vi "Read TC_PID.vi"(0 "read buffer":string, 11 "Error In":errorcluster) -> (4 "Temp (C)":dbl, 6 "On/Off Actual":bool, 8 "On/Off Set":bool, 10 "Temp Set Point (C)":i32, 13 "PID values":dbl[](array[numeric]), 14 "PWM":i32, 15 "Error Out":errorcluster)   [LabVIEW 2015]
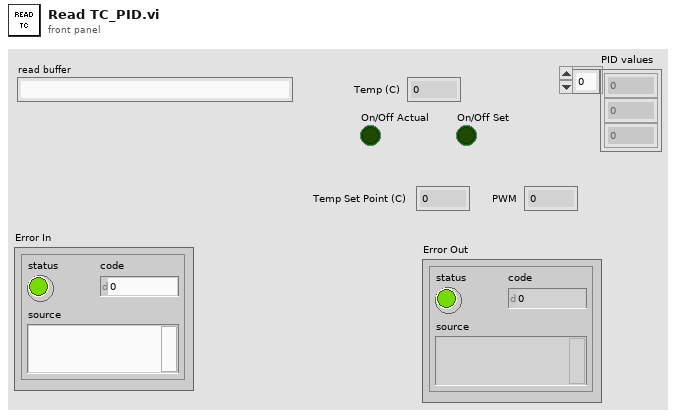
[diagram p1: front panel]
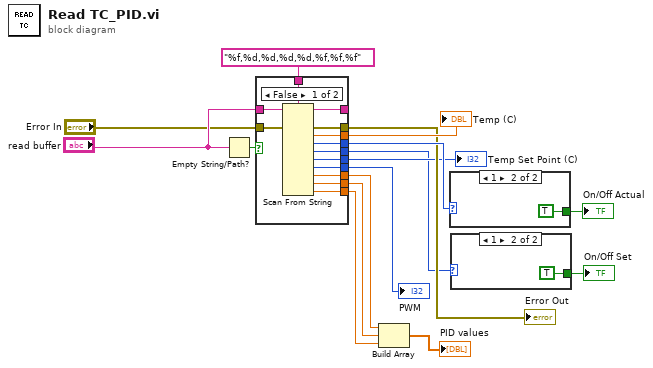
[diagram p0: block diagram]
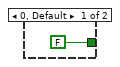
[diagram p2: hidden frame]
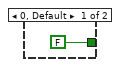
[diagram p3: hidden frame]
diagram:
  n1 = Empty String/Path?(string/path="read buffer") -> (empty?=w15:bool)
  n2 = case shown="False" w15 {
    tunnel: "read buffer" -> [w29 w31]
    tunnel: "%f,%d,%d,%d,%d,%f,%f,%f" ("format string") -> [w28 _]
    tunnel: [w27 w31] -> _
    tunnel: [w26 _] -> w13
    tunnel: [w25 _] -> w6
    tunnel: [w24 _] -> w12
    tunnel: [w23 w30] -> w10
    tunnel: "Error In" -> [w22 w30]
    tunnel: [w21 _] -> w7
    tunnel: [w20 _] -> w5
    tunnel: [w19 _] -> w4
    tunnel: [w18 _] -> w3
    tunnel: [w17 _] -> w2
    frame False {
      n3 = Scan From String(format string=w28, input string=w29, error in=w22) -> (remaining string=w27:string, error out=w23:errorcluster, output 1=w26:dbl, output 2=w24:i32, output 3=w25:i32, output 4=w21:i32, output 5=w20:i32, output 6=w19:dbl, output 7=w18:dbl, output 8=w17:dbl)  [unwired: 9 in, 1 out]
    }
    frame True {
    }
  }
  "Temp (C)" <- w13
  "Temp Set Point (C)" <- w7
  "Error Out" <- w10
  "PWM" <- w5
  n4 = Build Array(w4, w3, w2) -> (→"PID values":dbl[])
  n5 = case shown="1" w12 {
    tunnel: [FALSE TRUE] -> w11
    frame 0, Default {
    }
    frame 1 {
    }
  }
  "On/Off Actual" <- w11
  n6 = case shown="1" w6 {
    tunnel: [FALSE TRUE] -> w8
    frame 0, Default {
    }
    frame 1 {
    }
  }
  "On/Off Set" <- w8
